vi "words finder.vi"(7 "error in":errorcluster, 8 "bad expresion":string, 9 "good expresion":string, 10 "reference":refnum<visa-resource-name>) -> (0 "error out":errorcluster, 1 "bad state?":bool, 2 "response":string, 3 "reference out":refnum<visa-resource-name>)   [LabVIEW 2021]
panel:
  in  "delay":u32=50
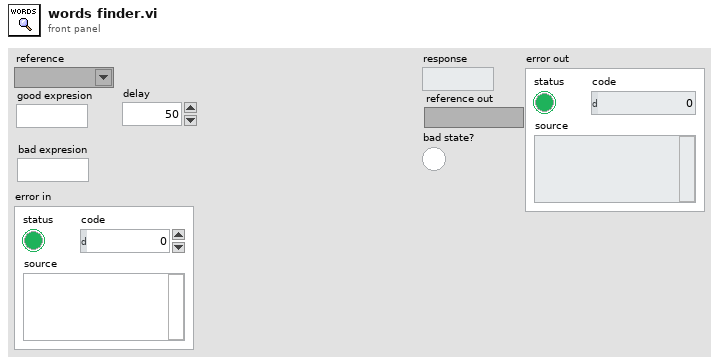
[diagram p1: front panel]
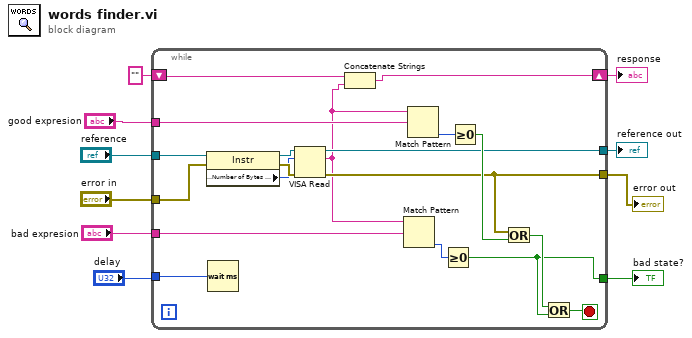
[diagram p0: block diagram]
diagram:
  n1 = while {
    tunnel: "reference" -> [w24]
    tunnel: "good expresion" -> [w23]
    shift-right: [w21] -> w7
    shift-left: "" -> [w22]
    tunnel: [w20] -> w6
    tunnel: "delay" -> [w19]
    tunnel: [w18] -> w3
    tunnel: "error in" -> [w17]
    tunnel: [w11] -> w2
    tunnel: "bad expresion" -> [w12]
    stop <- w16 stop-if-true
    n2 = property class="Instr"(reference=w24, error in=w17) -> (reference out=w27:refnum<visa-resource-name>, error out=w26:errorcluster, "Serial Settings:Number of Bytes at Serial Port"=w25:u32)
    n3 = Wait (ms)(milliseconds to wait=w19) -> ()  [unwired: 1 out]
    n4 = VISA Read(VISA resource name=w27, byte count=w25, error in (no error)=w26) -> (VISA resource name out=w20:refnum<visa-resource-name>, read buffer=w13:string, error out=w18:errorcluster)  [unwired: 1 out]
    n5 = Concatenate Strings(w22, w13) -> (w21:string)
    n6 = Match Pattern(string=w13, regular expression=w12) -> (offset past match=w14:i32)  [unwired: 1 in, 3 out]
    n7 = Match Pattern(string=w13, regular expression=w23) -> (offset past match=w29:i32)  [unwired: 1 in, 3 out]
    n8 = Greater Or Equal To 0?(x=w14) -> (x >= 0?=w11:bool)
    n9 = Greater Or Equal To 0?(x=w29) -> (x >= 0?=w28:bool)
    n10 = Or(x=w18, y=w28) -> (x .or. y?=w15:bool)
    n11 = Or(x=w15, y=w11) -> (x .or. y?=w16:bool)
  }
  "response" <- w7
  "reference out" <- w6
  "error out" <- w3
  "bad state?" <- w2
